vi "Untertitel change.vi"(8 "Fehler (Eingang, kein Fehler)":errorcluster, 9 "Sprachauswahl":u16, 10 "Sprachdatei":string[][](array[string]), 11 "Controls[]":refnum<vi>[](array[refnum])) -> (0 "Fehler (Ausgang, kein Fehler)":errorcluster caption="Fehler (Eingang, kein Fehler)", 2 "Sprachdatei out":string[][](array[string]), 3 "Untertiteln":string[](array[string]))   [LabVIEW 2020, in "Sprachverwaltung.lvlib"]
uses:
  Sprachverwaltung.lvlib
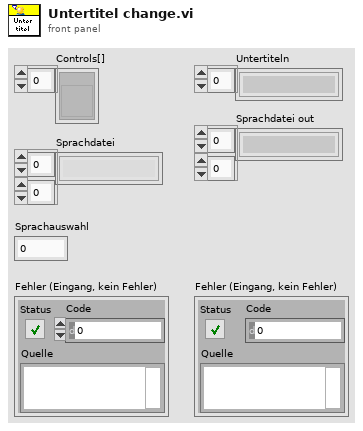
[diagram p1: front panel]
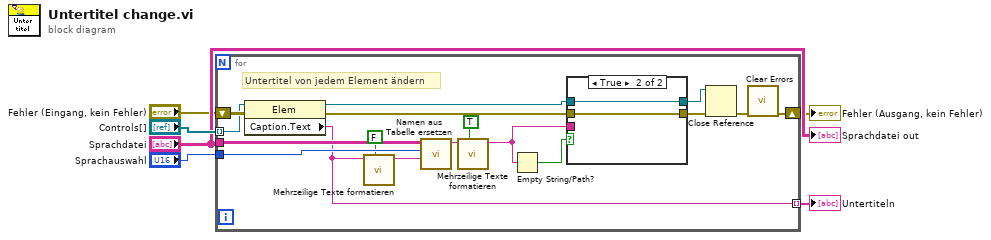
[diagram p0: block diagram]
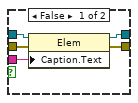
[diagram p2: hidden frame]
diagram:
  n1 = for {
    tunnel: "Sprachdatei" -> [w21]
    tunnel: "Controls[]" -> [w22] mode=indexing
    tunnel: "Sprachauswahl" -> [w20]
    tunnel: [w13] -> w6 mode=indexing
    shift-right: [w7] -> w1
    shift-left: "Fehler (Eingang, kein Fehler)" -> [_]
    # "Untertitel von jedem Element ändern"
    n2 = property class="Elem"(reference=w22) -> (reference out=w19:refnum<vi>, error out=w17:errorcluster, "Caption.Text"=w13:string)  [unwired: 1 in]
    n3 = call "Mehrzeilige Texte formatieren.vi"("Zurück formatieren"=FALSE, "string"=w13) -> ("result string"=w12:string)  [unwired: 9 in]
    n4 = call "Namen aus Tabelle ersetzen.vi"("Regulärer Ausdruck"=w12, "Sprachauswahl"=w20, "Tabelle"=w21) -> ("Übersetzung"=w10:string)  [unwired: 7 in, 1 out]
    n5 = call "Mehrzeilige Texte formatieren.vi"("Zurück formatieren"=TRUE, "string"=w10) -> ("result string"=w9:string)  [unwired: 9 in]
    n6 = Empty String/Path?(string/path=w9) -> (empty?=w18:bool)
    n7 = case shown="True" w18 {
      tunnel: w19 -> [w27 w29]
      tunnel: w17 -> [w26 w28]
      tunnel: [w25 w29] -> w15
      tunnel: [w24 w28] -> w14
      tunnel: w9 -> [w23 _]
      frame False {
        n8 = property class="Elem"(reference=w27, error in=w26, "Caption.Text"=w23) -> (reference out=w25:refnum<vi>, error out=w24:errorcluster)
      }
      frame True {
      }
    }
    n9 = Close Reference(reference=w15, error in (no error)=w14) -> (error out=w16:errorcluster)
    n10 = call <vilib>:"Clear Errors.vi"("error in (no error)"=w16) -> ("error out"=w7:errorcluster)  [unwired: 5 in, 1 out]
  }
  "Untertiteln" <- w6
  "Fehler (Ausgang, kein Fehler)" <- w1
  "Sprachdatei out" <- "Sprachdatei"
